vi "GetSpeed.vi"(5 "Max Window":dbl=1800.0 format="%.4f", 7 "Min Window":dbl=300.0 format="%.4f", 8 "error in (no error)":errorcluster, 9 "Y":dbl[](array[numeric]), 11 "comm seg":dbl=2.0) -> (0 "error out":errorcluster, 3 "Speed":dbl)   [LabVIEW 2013]
uses:
  <vilib>/addons/Spectral Measurements Toolset/LVSupport/SMT Zoom Power Spectrum (WDT).vi
  <vilib>/addons/Spectral Measurements Toolset/niSMT.lvlib
panel:
  in  "advanced settings":T1={"window"=enum."7 Term B-Harris", "spectral lines"=-1, "effective band specification"={"fl"=0.0, "fh"=0.5}, "RBW definition"=enum."3dB"} {"effective band specification"."fh" format="%.2f"; "effective band specification"."fl" format="%.2f"}
  in  "spectrum settings":T2={"center frequency"=12000000.0, "span"=5000000.0, "resolution bandwidth"=-1.0} {"resolution bandwidth" format="%.2p"; "center frequency" format="%.2p"; "span" format="%.2p"}
  in  "averaging parameters":T3={"averaging type"=enum."no averaging", "averaging settings"={"weighting type"=enum."exponential", "weighting settings"={"size"=1.0, "linear weighting mode"=enum."moving average"}}}
  in  "peak search settings":T4={"single/multiple"=enum."Single Max Peak", "threshold"=0.01} {"threshold" format="%.2f"}
  in  "unit conversion settings":T5={"units"=enum."V", "peak scaling"=enum."rms", "psd?"=FALSE, "impedance(ohm)"=50.0} {"impedance(ohm)" format="%.2f"}
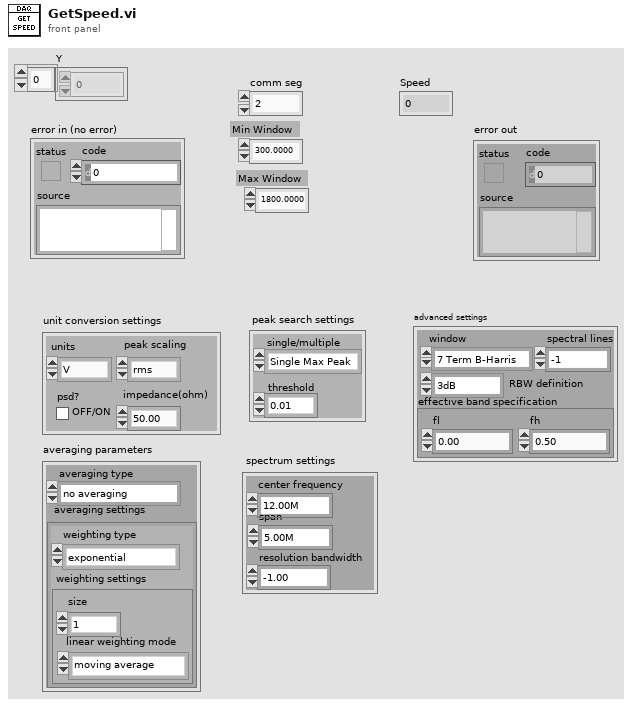
[diagram p1: front panel]
types:
  T1 = cluster{"window":enum16{"None ", "Hanning", "Hamming", "Blackman-Harris", "Exact Blackman", "Blackman", "Flat Top", "4 Term B-Harris ", "7 Term B-Harris", "Low Sidelobe"}, "spectral lines":i32, "effective band specification":cluster{"fl":dbl, "fh":dbl}, "RBW definition":enum16{"3dB", "6dB", "ENBW", "bin width"}}
  T2 = cluster{"center frequency":dbl, "span":dbl, "resolution bandwidth":dbl}
  T3 = cluster{"averaging type":enum16{"no averaging", "vector averaging", "RMS averaging", "peak hold"}, "averaging settings":cluster{"weighting type":enum16{"linear", "exponential"}, "weighting settings":cluster{"size":dbl, "linear weighting mode":enum16{"one shot", "auto restart one shot", "moving average", "continuous"}}}}
  T4 = cluster{"single/multiple":enum16{"Multiple Peaks", "Single Max Peak"}, "threshold":dbl}
  T5 = cluster{"units":enum16{"V", "V^2", "W", "dBm", "dBW", "dBV", "dBmV", "dBuV"}, "peak scaling":enum16{"rms", "pk"}, "psd?":bool, "impedance(ohm)":dbl}
  T6 = cluster{"type":enum16{"real", "complex modulated"}, "frequency shift":dbl}
  T7 = typedef "niSMT.lvlib/SMT zoom settings.ctl" = cluster{"zoom FFT settings":T8, "frequency shift":dbl, "data format":enum16{"real", "complex modulated (array)", "complex modulated (interleaved)"}}
  T8 = typedef "NI_MAPro.lvlib/ma_sml_ND Zoom FFT Settings.ctl" = cluster{"zoom settings":cluster{"center frequency":dbl, "zoom":i32, "trim":dbl}, "FFT settings":cluster{"window":u16, "FFT size":i32}}
  T9 = typedef "NI_MAPro.lvlib/ma_sml_Spectral Info.ctl" = cluster{"spectrum type":enum16{"FFT Spectrum [complex]", "Amplitude [Magnitude]", "Power [Magnitude^2]", "Cross Spectrum [complex]", "Frequency Response [Complex]"}, "linear/dB":enum16{"linear", "dB"}, "window":u16, "window size":i32, "FFT size":i32}
  T10 = typedef "NI_MAPro.lvlib/ma_sml_Spectrum Cluster (real).ctl" = cluster{"f0":dbl, "df":dbl, "spectrum":dbl[]}
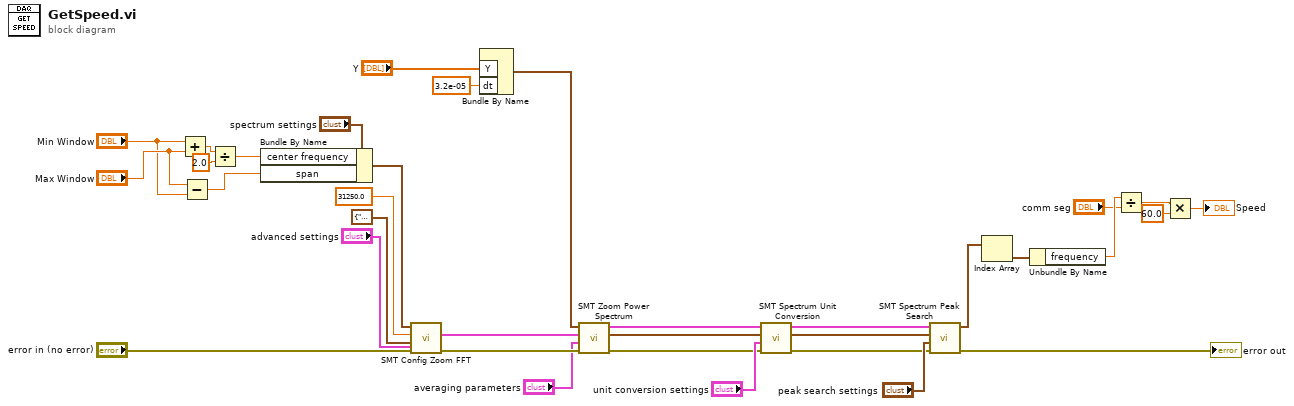
[diagram p0: block diagram]
diagram:
  n1 = Add(x="Min Window", y="Max Window") -> (x+y=w24:dbl)
  n2 = Subtract(x="Max Window", y="Min Window") -> (x-y=w26:dbl)
  n3 = Divide(x=w24, y=2.0) -> (x/y=w22:dbl)
  n4 = Bundle By Name(cluster="spectrum settings", "center frequency"=w22, "span"=w26) -> (w27:T2)
  n5 = call <vilib>:"SMT Config Zoom FFT.vi"("advanced settings"="advanced settings", "error in (no error)"="error in (no error)", "input signal settings"=T6 {"type"=enum."real", "frequency shift"=0.0}, "fs"=31250.0, "spectrum settings"=w27) -> ("error out"=w19:errorcluster, "SMT zoom settings"=w18:T7)  [unwired: 3 in, 2 out]
  n6 = Bundle By Name("Y"="Y", "dt"=3.2e-05) -> (w4:waveform(dbl))  [unwired: 1 in]
  n7 = call-poly <vilib>:"SMT Zoom Power Spectrum.vi"("error in (no error)"=w19, "averaging parameters"="averaging parameters", "SMT zoom settings"=w18, "signal in"=w4) -> ("error out"=w14:errorcluster, "spectral info"=w13:T9, "power spectrum"=w1:T10)  [unwired: 3 in, 2 out]
  n8 = call <vilib>:"SMT Spectrum Unit Conversion.vi"("error in (no error)"=w14, "unit conversion settings"="unit conversion settings", "spectral info in"=w13, "power spectrum"=w1) -> ("error out"=w12:errorcluster, "spectral info out"=w11:T9, "unit converted spectrum"=w3:cluster{"f0":dbl, "df":dbl, "spectrum":dbl[]})  [unwired: 4 in, 1 out]
  n9 = call <vilib>:"SMT Spectrum Peak Search.vi"("error in (no error)"=w12, "peak search setting"="peak search settings", "spectral info"=w11, "power spectrum"=w3) -> ("error out"=→"error out":errorcluster, "peaks"=w9:cluster{"frequency":dbl, "value":dbl}[])  [unwired: 5 in, 1 out]
  n10 = Index Array(array=w9) -> (element=w28:cluster{"frequency":dbl, "value":dbl})  [unwired: 1 in]
  n11 = Unbundle By Name(w28) -> ("frequency"=w10:dbl)
  n12 = Divide(x=w10, y="comm seg") -> (x/y=w29:dbl)
  n13 = Multiply(x=w29, y=60.0) -> (x*y=→"Speed":dbl)
